vi "Create (Factory).vi"(5 "Sequencer":refnum<class "MessageQ.lvclass">, 6 "Variables":refnum<class "Variables.lvclass">, 7 "VolatusAPI":refnum<class "VolatusAPI.lvclass">, 8 "error in (no error)":refnum<class "MultiErrors.lvclass">, 10 "Command Config":refnum<class "Command Config.lvclass">) -> (0 "error out":refnum<class "MultiErrors.lvclass">, 3 "Command":T1)   [LabVIEW 2020, in "VolatusSeq.lvlib" / "Command.lvclass"]
uses:
  Command.lvclass
  Command.lvclass/Command.ctl
  VolatusSeq.lvlib
  VolatusErrorUtilities/MultiErrors/MultiErrors.lvclass
  VolatusSeqConfig/Command Config/Command Config.lvclass
  Volatus/VolatusAPI/VolatusAPI.lvclass
  VolatusSeqConfig/Command Type.ctl
  VolatusSeqConfig/VolatusSeqConfig.lvlib
  Volatus/MessageQ/MessageQ.lvclass
  Command.ctl
  messages/CmdDigital/Data.ctl
  messages/CmdDigital/CmdDigital.lvlib
  messages/CmdAnalog/Data.ctl
  messages/CmdAnalog/CmdAnalog.lvlib
  Send Type.ctl
  Variables/Variables.lvclass
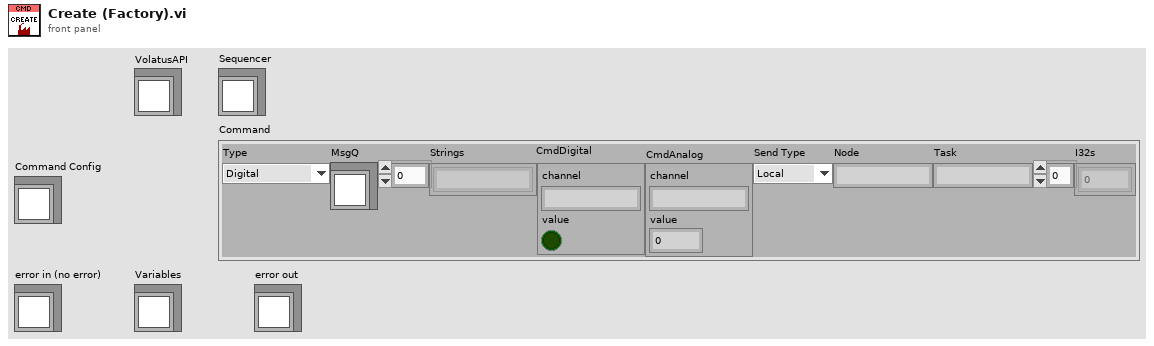
[diagram p1: front panel]
types:
  T1 = typedef "VolatusSeq.lvlib/Command.ctl" = cluster{"Type":T2, "MsgQ":refnum<class "MessageQ.lvclass">, "Strings":string[], "CmdDigital":T3, "CmdAnalog":T4, "Send Type":T5, "Node":string, "Task":string, "I32s":i32[]}
  T2 = typedef "VolatusSeqConfig.lvlib/Command Type.ctl" = enum16{"Digital", "Numeric", "Transition", "Stop", "StartLog", "StopLog", "Start", "Event", "Error", "HTTP", "ResetVar", "IncVar", "DecVar", "SaveVar", "LoadVar", "AddVar", "SubVar"}
  T3 = typedef "CmdDigital.lvlib/Data.ctl" = cluster{"channel":string, "value":bool}
  T4 = typedef "CmdAnalog.lvlib/Data.ctl" = cluster{"channel":string, "value":dbl}
  T5 = typedef "VolatusSeq.lvlib/Send Type.ctl" = enum16{"Local", "Remote"}
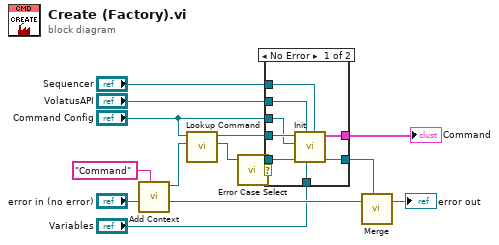
[diagram p0: block diagram]
diagram:
  n1 = call "Add Context.vi"("Context"="Command", "MultiErrors in"="error in (no error)") -> ("Original Context"=w11:refnum<class "MultiErrors.lvclass">, "Added Context"=w10:refnum<class "MultiErrors.lvclass">)  [unwired: 8 in]
  n2 = call "Lookup Command.vi"("error in (no error)"=w10, "Command Config"="Command Config") -> ("error out"=w8:refnum<class "MultiErrors.lvclass">, "Command"=w14:refnum<class "Command.lvclass">)  [unwired: 8 in]
  n3 = call "Error Case Select.vi"("MultiErrors in"=w8) -> ("MultiErrors out"=w7:refnum<class "MultiErrors.lvclass">, "error out"=w6:errorcluster)  [unwired: 7 in]
  n4 = case shown="No Error" w6 {
    tunnel: "VolatusAPI" -> [w22 _]
    tunnel: w14 -> [w23 _]
    tunnel: "Command Config" -> [w21 _]
    tunnel: w7 -> [w20 w24]
    tunnel: [w18 w24] -> w4
    tunnel: [w19 _] -> w3
    tunnel: "Sequencer" -> [w17 _]
    tunnel: "Variables" -> [w16 _]
    frame No Error {
      n5 = call "Init.vi"("Sequencer"=w17, "Variables"=w16, "VolatusAPI"=w22, "error in (no error)"=w20, "Command Config"=w21, "Command in"=w23) -> ("error out"=w18:refnum<class "MultiErrors.lvclass">, "Command"=w19:T1)  [unwired: 4 in]
    }
    frame Error {
    }
  }
  "Command" <- w3
  n6 = call "Merge.vi"("First Error In"=w11, "Second Error In"=w4) -> ("MultiErrors out"=→"error out":refnum<class "MultiErrors.lvclass">)  [unwired: 5 in]
